vi "PLAN_CREATOR.vi"(8 "error In":errorcluster) -> (0 "error out":errorcluster)   [LabVIEW 2017]
uses:
  Controls/Ass. Loop Control.ctl
  <vilib>/Utility/error.llb/DialogType.ctl
panel:
  in  "PLAN NAME":string(combo)
  in  "CURRENT PLAN TABLE":string[][](table)
  in  "REMOVE PART":bool
  in  "ADD PART":bool
  in  "LIST OF PARTS":string(combo)
  in  "DOORS":string(combo)
  out "USER:-":string
  in  "Stop":bool
  out "DATE/TIME":string
  out "Screen Name":string
  # "Nm"
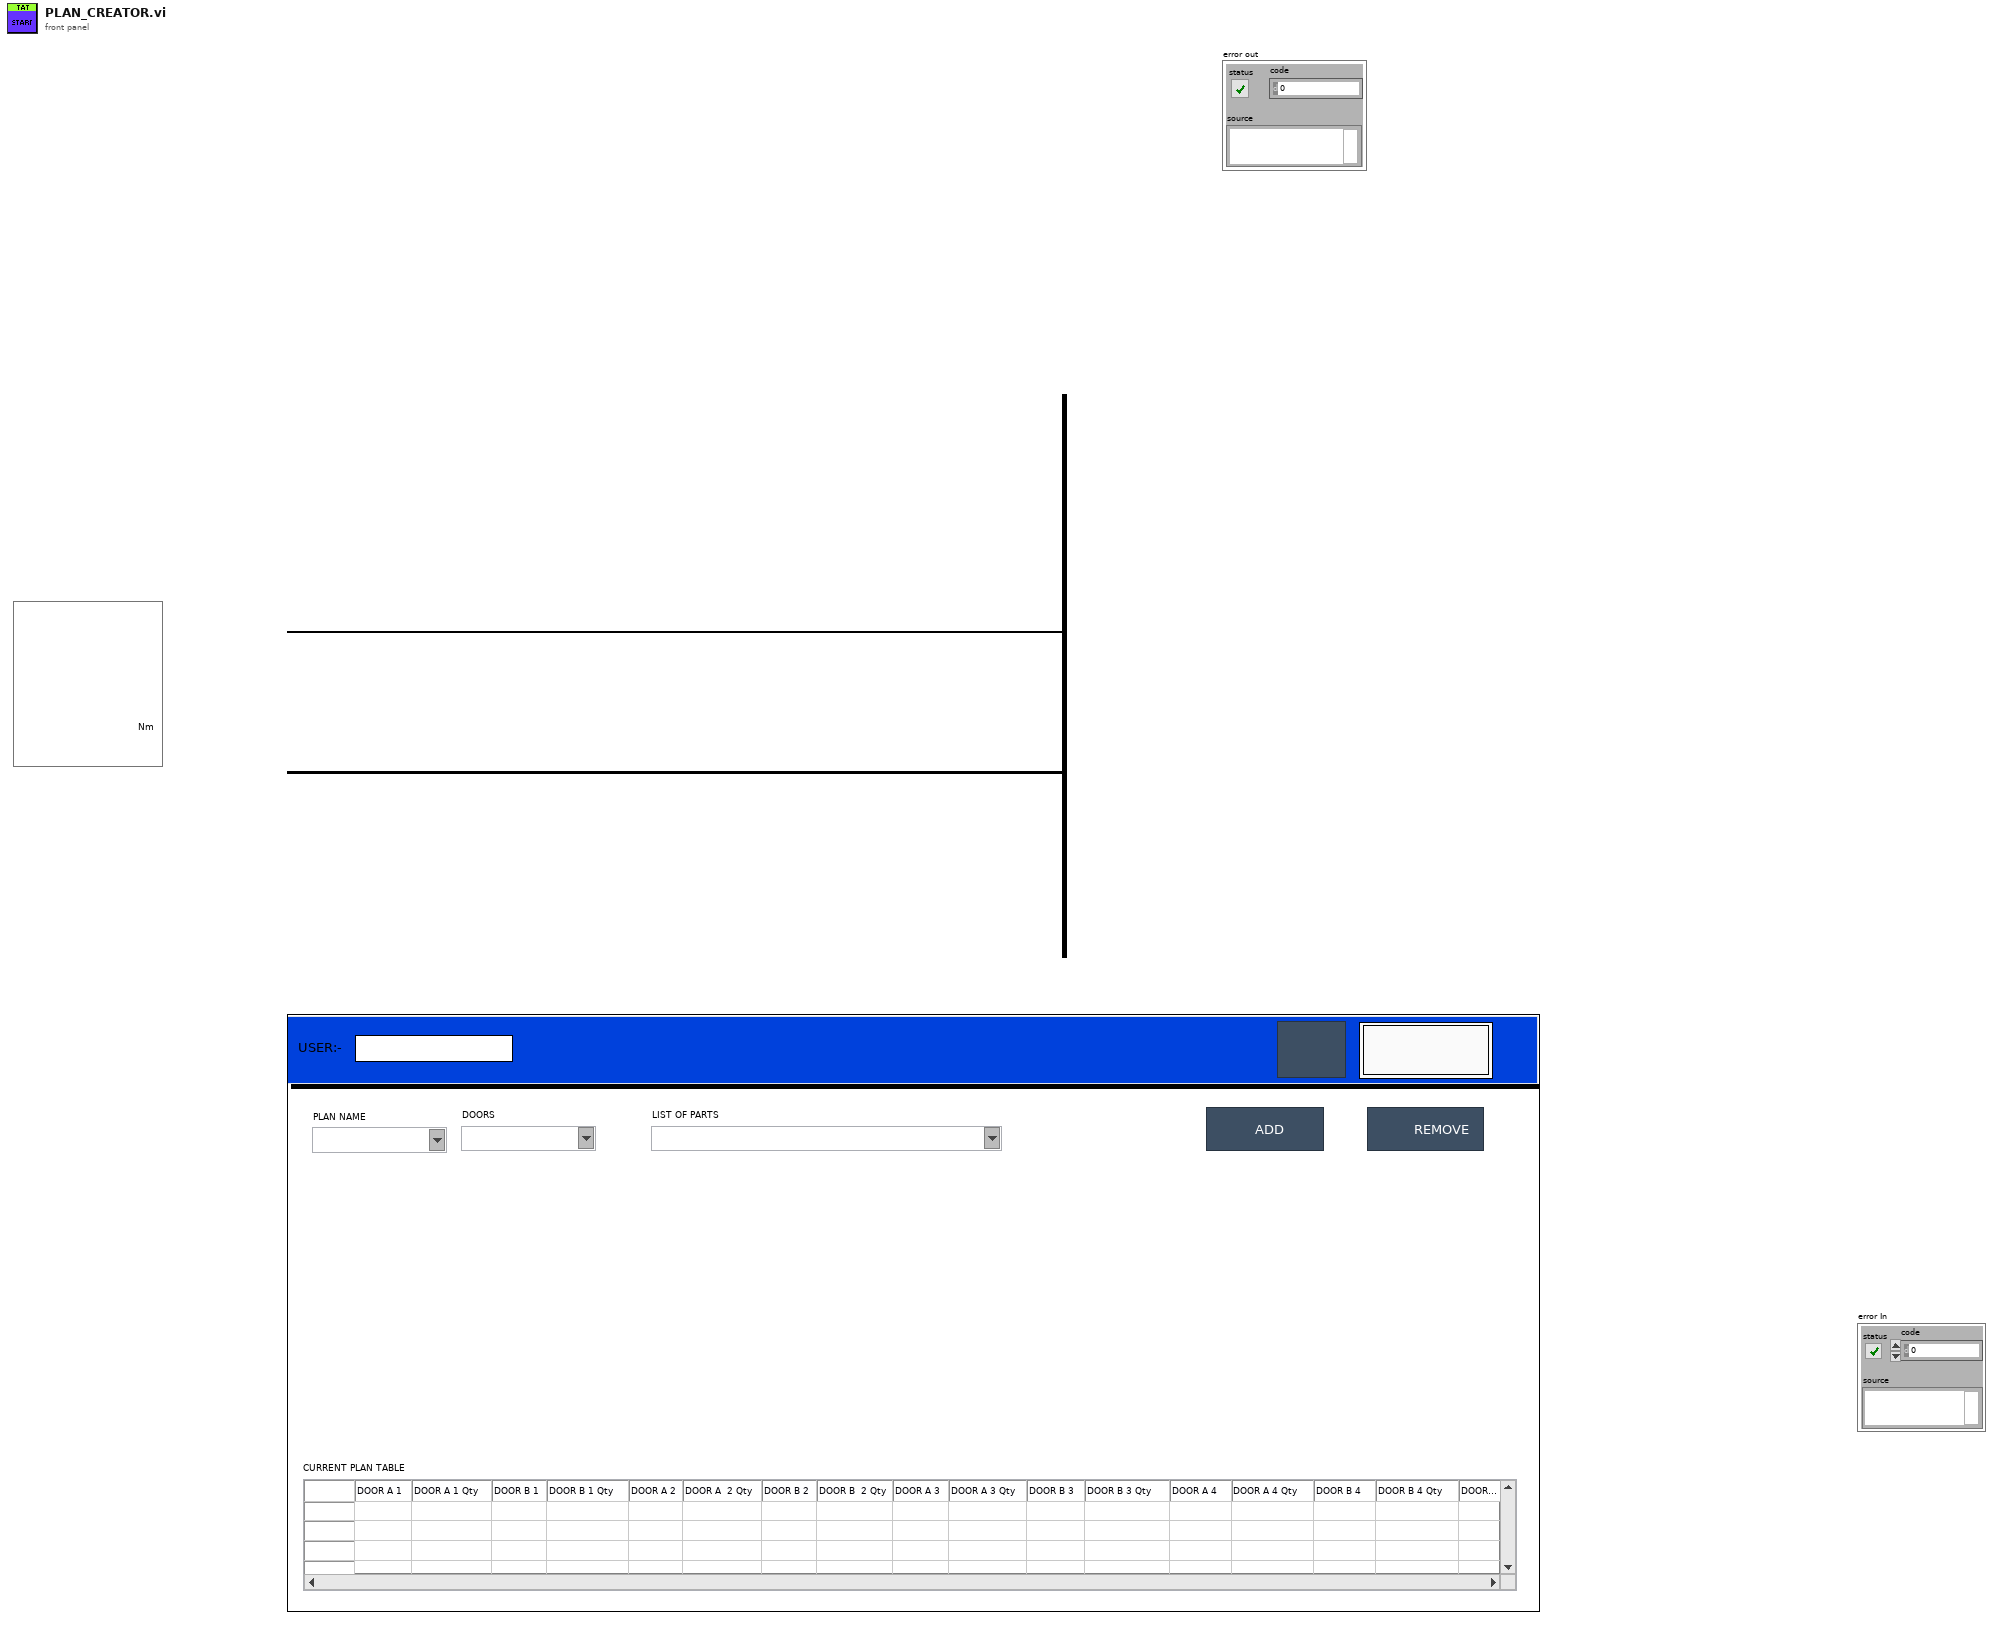
[diagram p1: front panel]
types:
  T1 = typedef "DialogType.ctl" = u16
  T2 = typedef "Ass. Loop Control.ctl" = enum16{"Package_Qty_Count", "GENERATE_QR_PRNT", "Cluster_update", "Waiting_for_scan", "barcode CHECK", "Int", "SaveReport ", "Barcode Print", "Start Cycle", "Wait", "Cycle End", "Stop"}
  T3 = enum32{"invalid app kind", "Development System", "Run Time System", "Student Edition", "Embedded LabVIEW", "Evaluation", "Custom"}
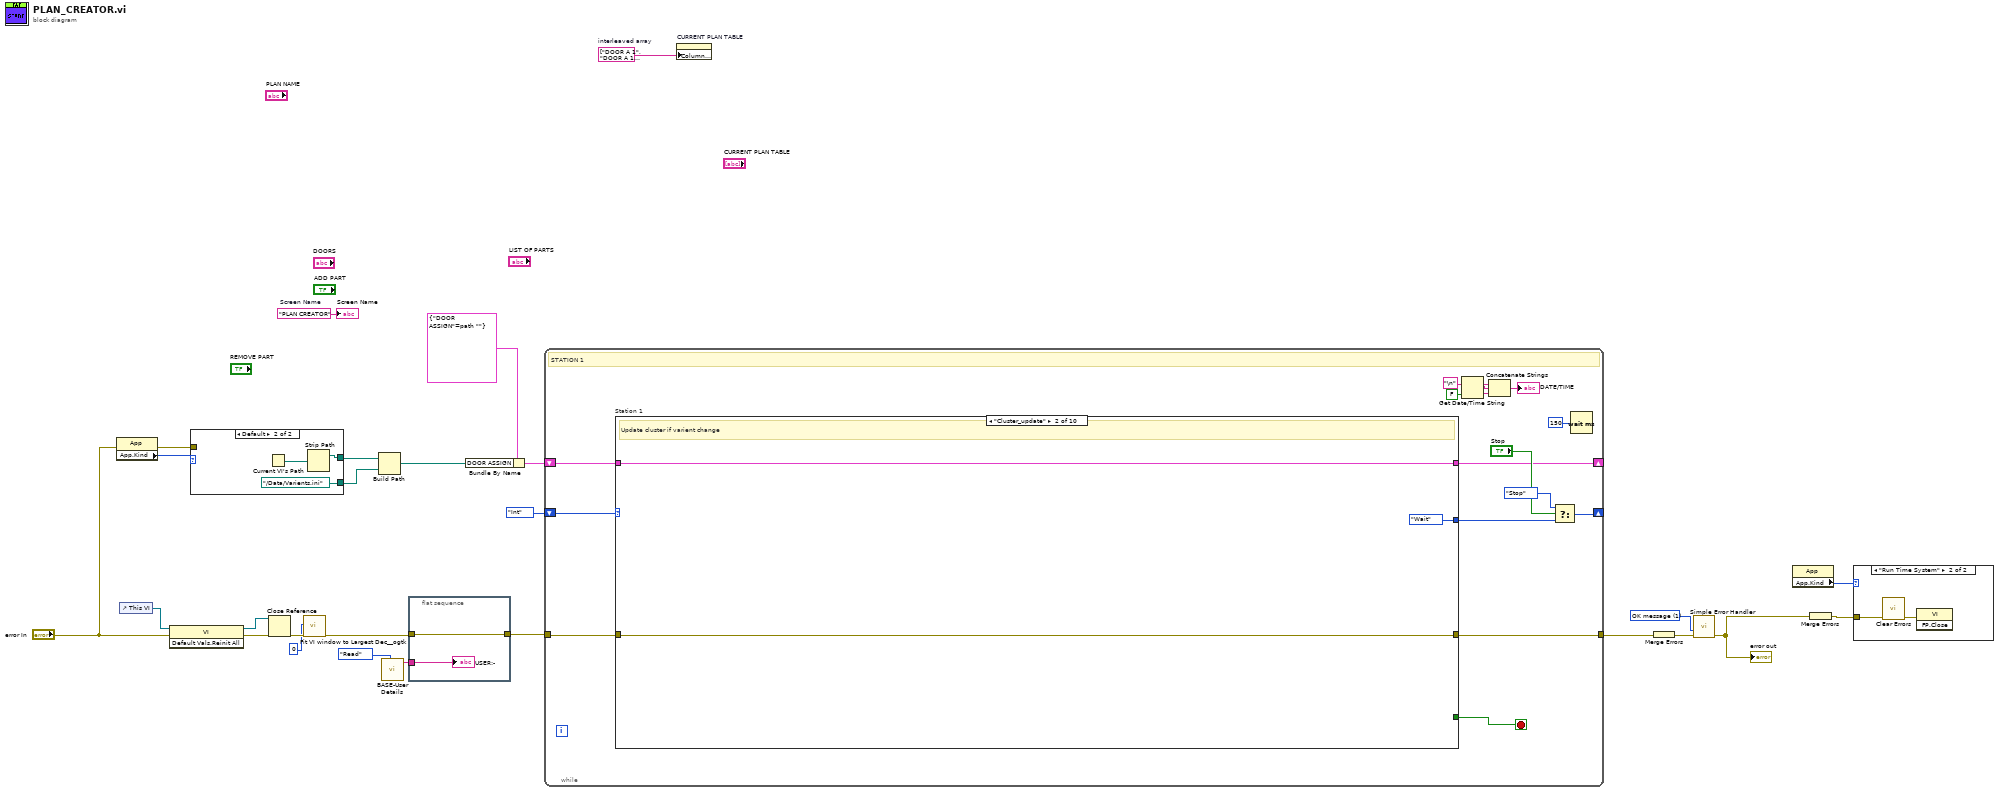
[diagram p0: block diagram]
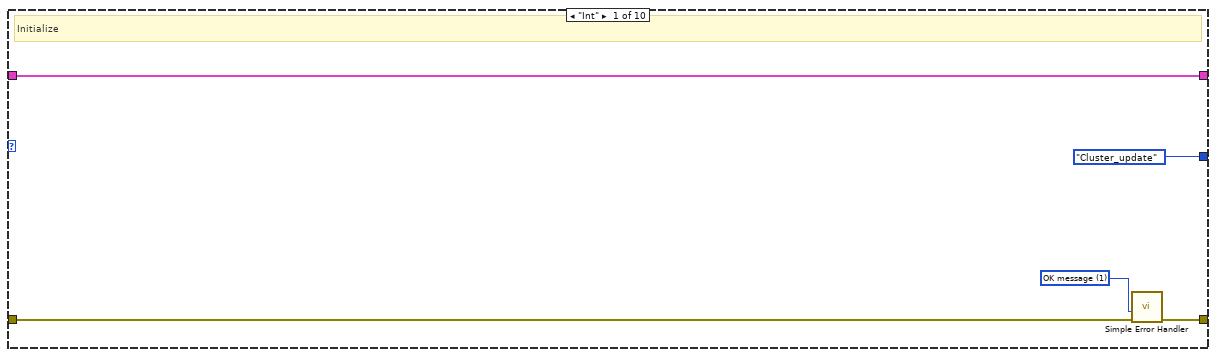
[diagram p3: hidden frame]
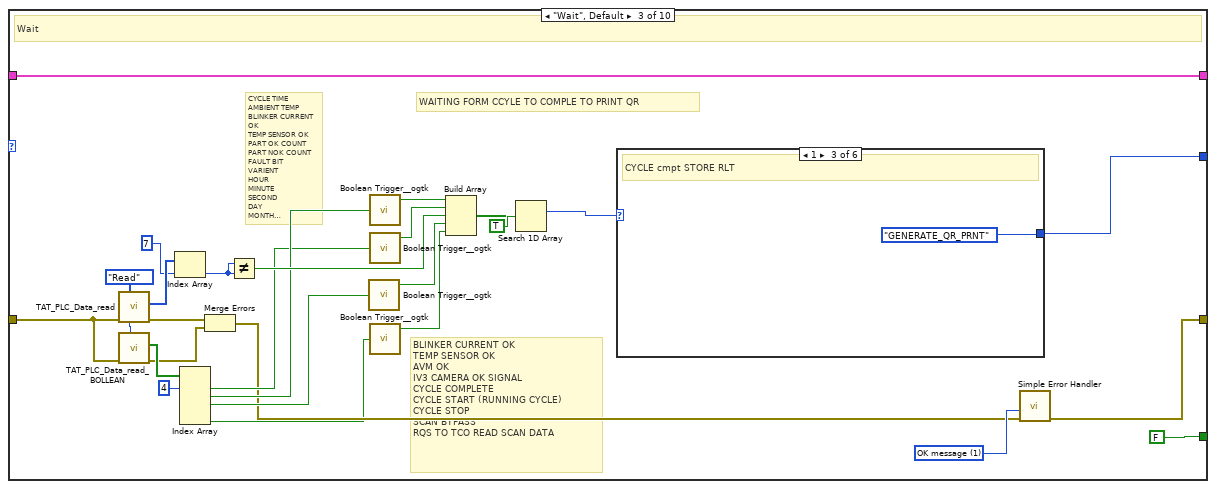
[diagram p4: hidden frame]
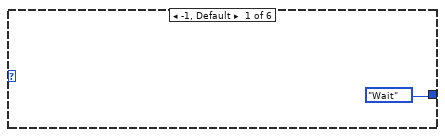
[diagram p5: hidden frame]
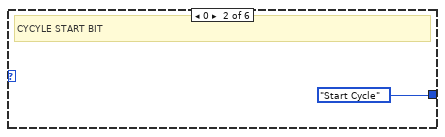
[diagram p6: hidden frame]
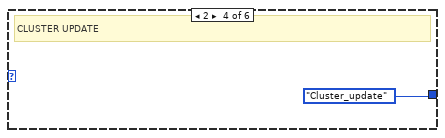
[diagram p7: hidden frame]
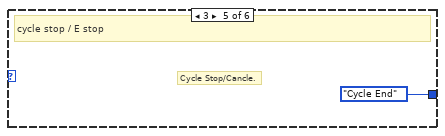
[diagram p8: hidden frame]
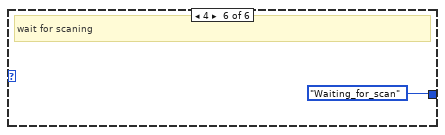
[diagram p9: hidden frame]
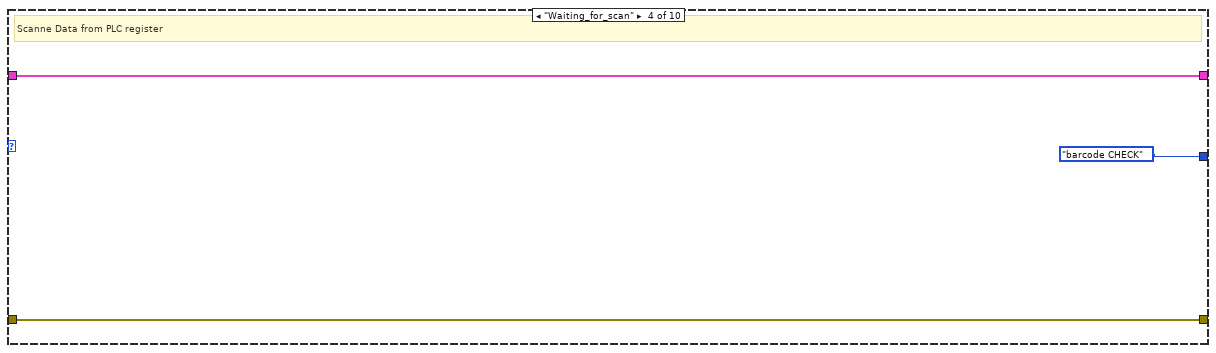
[diagram p10: hidden frame]
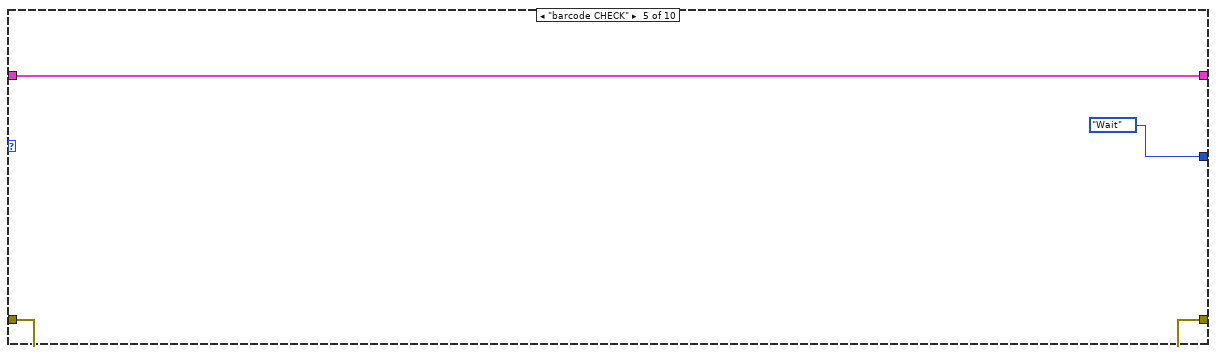
[diagram p11: hidden frame]
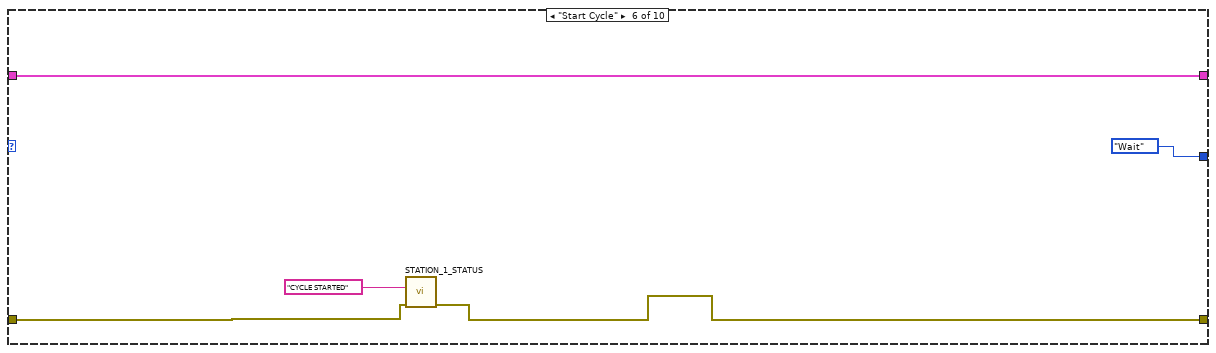
[diagram p12: hidden frame]
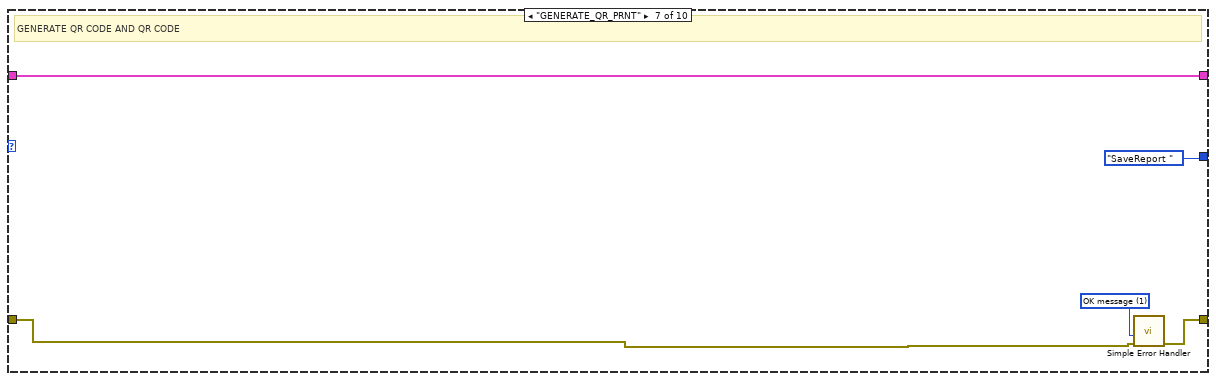
[diagram p13: hidden frame]
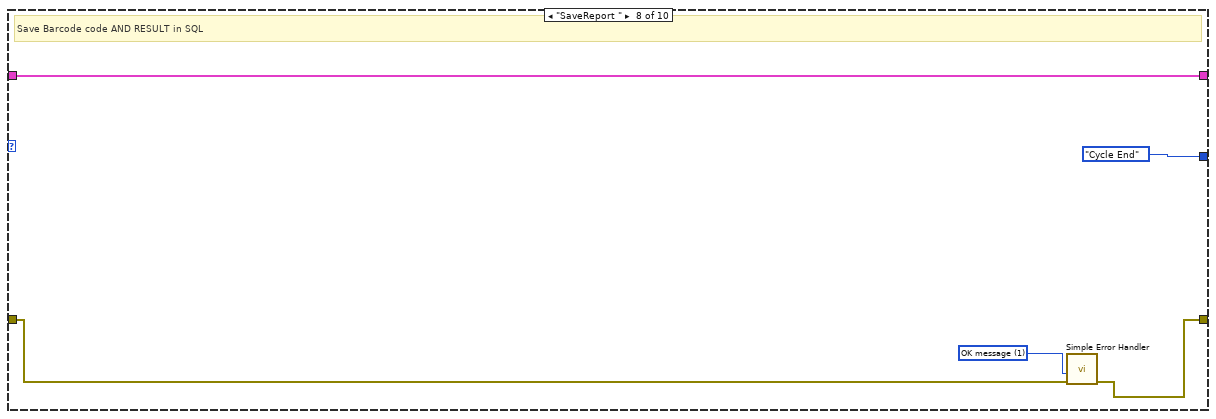
[diagram p14: hidden frame]
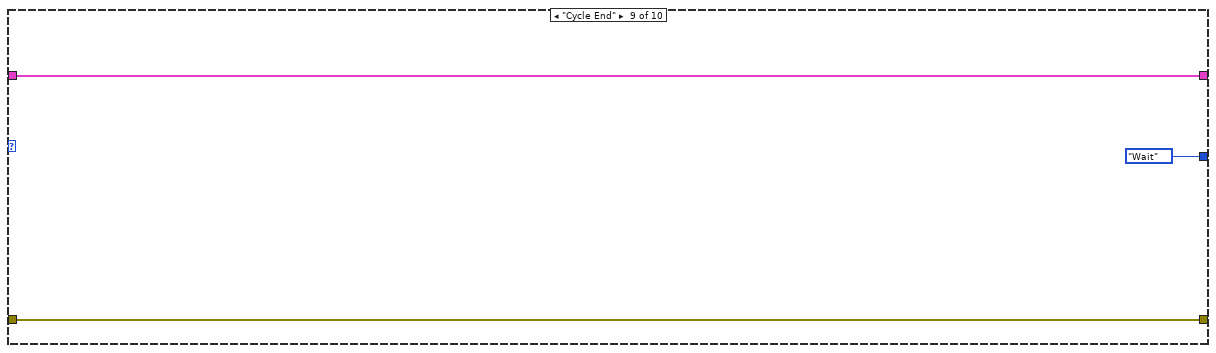
[diagram p15: hidden frame]
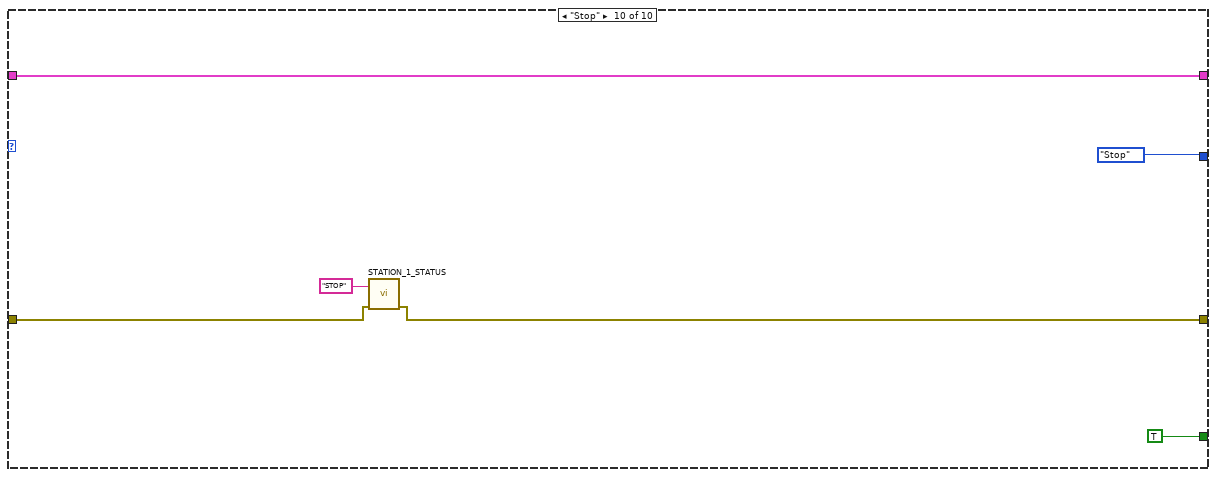
[diagram p16: hidden frame]
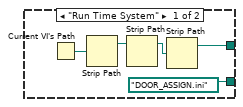
[diagram p17: hidden frame]
diagram:
  w1 = string[] ["DOOR A 1", "DOOR A 1 Qty", "DOOR B 1", "DOOR B 1 Qty", "DOOR A 2", "DOOR A  2 Qty", "DOOR B 2", "DOOR B  2 Qty", "DOOR A 3", "DOOR A 3 Qty", "DOOR B 3", "DOOR B 3 Qty", "DOOR A 4", "DOOR A 4 Qty", "DOOR B 4", "DOOR B 4 Qty", "DOOR A 5", "DOOR A 5 Qty", "DOOR B 5", "DOOR B 5 Qty", "DOOR A 11", "DOOR A 11 Qty", "DOOR B 11", "DOOR B 11 Qty", "DOOR A 12", "DOOR A 12 Qty", "DOOR B 12", "DOOR B 12 Qty", "DOOR A 13", "DOOR A 13 Qty", "DOOR B 13", "DOOR B 13 Qty", "DOOR A 14", "DOOR A 14 Qty", "DOOR B 14", "DOOR B 14 Qty", "DOOR A 15", "DOOR A 15 Qty", "DOOR B 15", "DOOR B 15 Qty", "DOOR A 16", "DOOR A 16 Qty", "DOOR B 16", "DOOR B 16 Qty"]  # interleaved array
  w5 = "PLAN CREATOR"  # Screen Name
  w17 = T1 1 items=["no dialog", "OK message", "continue or stop message", "OK message + warnings", "continue/stop + warnings"] ("type of dialog (OK msg:1)")
  n1 = property class="App"(error in="error In") -> (error out=w13:errorcluster, "App.Kind"=w15:T3)  [unwired: 1 in, 1 out]
  n2 = control-ref of="This VI"() -> (w26:refnum<vi>)
  n3 = invoke class="VI" method="Default Vals.Reinit All"(reference=w26, error in="error In") -> (reference out=w24:refnum<vi>, error out=w25:errorcluster)  [unwired: 1 in, 1 out]
  n4 = case shown="Default" w15 {
    tunnel: [path "DOOR_ASSIGN.ini" ("path") path "../Data/Varients.ini" ("path")] -> w14
    tunnel: [w27 w32] -> w7
    tunnel: w13 -> [_ _]
    frame "Run Time System" {
      n5 = Current VI's Path() -> (path=w30:path)
      n6 = Strip Path(path=w30) -> (stripped path=w29:path)  [unwired: 1 out]
      n7 = Strip Path(path=w29) -> (stripped path=w28:path)  [unwired: 1 out]
      n8 = Strip Path(path=w28) -> (stripped path=w27:path)  [unwired: 1 out]
    }
    frame Default {
      n9 = Current VI's Path() -> (path=w33:path)
      n10 = Strip Path(path=w33) -> (stripped path=w32:path)  [unwired: 1 out]
    }
  }
  n11 = Close Reference(reference=w24, error in (no error)=w25) -> (error out=w23:errorcluster)
  n12 = call <userlib>:"Fit VI window to Largest Dec__ogtk.vi"("error in (no error)"=w23, "border spacing (2 px)"=0) -> ("error out"=w11:errorcluster)  [unwired: 4 in, 1 out]
  n13 = Build Path(base path=w7, name or relative path=w14) -> (appended path=w3:path)
  n14 = call "BASE-User Details.vi"("Enum"=enum16{"Read", "Write"}."Read") -> ("User Name Out"=w18:string)  [unwired: 9 in, 1 out]
  n15 = flat-sequence {
    tunnel: [w36] -> w6
    tunnel: w11 -> [w36]
    tunnel: w18 -> [w35]
    frame #0 {
      "USER:-" <- w35
    }
  }
  n16 = Bundle By Name(cluster=cluster{"DOOR ASSIGN":path} {"DOOR ASSIGN"=path ""}, "DOOR ASSIGN"=w3) -> (w2:cluster{"DOOR ASSIGN":path})
  n17 = while {
    tunnel: w6 -> [w39]
    shift-right: [w49] -> _
    shift-left: Ass._Loop_Control."Int" ("Enum") -> [w52]
    tunnel: [w50] -> w21
    shift-right: [w37] -> _
    shift-left: w2 -> [w38]
    stop <- w42 stop-if-true
    # "STATION 1"
    n18 = case "Station 1" shown="\"Cluster_update\"" w52 {
      tunnel: [Ass._Loop_Control."Cluster_update" ("Enum") Ass._Loop_Control."Wait" ("Enum") w81 Ass._Loop_Control."barcode CHECK" ("Enum") Ass._Loop_Control."Wait" ("Enum") Ass._Loop_Control."Wait" ("Enum") Ass._Loop_Control."SaveReport " ("Enum") Ass._Loop_Control."Cycle End" ("Enum") Ass._Loop_Control."Wait" ("Enum") Ass._Loop_Control."Stop" ("Enum")] -> w41
      tunnel: [_ _ FALSE _ _ _ _ _ _ TRUE] -> w42
      tunnel: [w55 w59 w78 w95 w98 w101 w108 w112 w116 w119] -> w50
      tunnel: w39 -> [w54 w59 w75 w95 w98 w102 w106 w111 w116 w120]
      tunnel: w38 -> [w53 w58 w61 w94 w97 w100 w105 w110 w115 w118]
      tunnel: [w53 w58 w61 w94 w97 w100 w105 w110 w115 w118] -> w37
      frame "Int" {
        w56 = T1 1 items=["no dialog", "OK message", "continue or stop message", "OK message + warnings", "continue/stop + warnings"] ("type of dialog (OK msg:1)")
        # "Initialize"
        n19 = call <vilib>:"Simple Error Handler.vi"("type of dialog (OK msg:1)"=w56, "error in (no error)"=w54) -> ("error out"=w55:errorcluster)  [unwired: 3 in, 4 out]
      }
      frame "Cluster_update" {
        # "Update cluster if varient change"
      }
      frame "Wait", Default {
        w79 = T1 1 items=["no dialog", "OK message", "continue or stop message", "OK message + warnings", "continue/stop + warnings"] ("type of dialog (OK msg:1)")
        w76 = enum16{"Read", "Write"}."Read" ("Enum")
        # "CYCLE TIME\nAMBIENT TEMP\nBLINKER CURRENT OK\nTEMP SENSOR OK\nPART OK COUNT\nPART NOK COUNT\nFAULT BIT\nVARIENT\nHOUR\nMINUTE\nSECOND\nDAY\nMONTH\nYEAR\nSERIAL NUMBER"
        # "BLINKER CURRENT OK\nTEMP SENSOR OK\nAVM OK\nIV3 CAMERA OK SIGNAL\nCYCLE COMPLETE\nCYCLE START (RUNNING CYCLE)\nCYCLE STOP\nSCAN BYPASS\nRQS TO TCO READ SCAN DATA"
        # "WAITING FORM CCYLE TO COMPLE TO PRINT QR"
        # "Wait"
        n20 = call "TAT_PLC_Data_read.vi"("Enum"=w76, "error in (no error)"=w75) -> ("error out"=w66:errorcluster, "Array 2"=w82:u16[])  [unwired: 8 in]
        n21 = call "TAT_PLC_Data_read_BOLLEAN.vi"("Enum"=w76, "error in (no error)"=w75) -> ("error out"=w64:errorcluster, "Array 2"=w74:bool[])  [unwired: 8 in]
        n22 = Index Array(array=w82, index=7) -> (element=w62:u16)
        n23 = Index Array(array=w74, index #1=4 ("index")) -> (element #1=w71:bool, element #2=w72:bool, element #3=w70:bool, element #5=w63:bool)  [unwired: 4 in, 1 out]
        n24 = Merge Errors(w66, w64) -> (w65:errorcluster)
        n25 = Not Equal?(x=w62, y=w62) -> (x != y?=w80:bool)
        n26 = call <userlib>:"Boolean Trigger__ogtk.vi"("Boolean Input"=w70) -> ("Rising Edge"=w69:bool)  [unwired: 1 in, 1 out]
        n27 = call <userlib>:"Boolean Trigger__ogtk.vi"("Boolean Input"=w72) -> ("Rising Edge"=w86:bool)  [unwired: 1 in, 1 out]
        n28 = call <userlib>:"Boolean Trigger__ogtk.vi"("Boolean Input"=w71) -> ("Rising Edge"=w77:bool)  [unwired: 1 in, 1 out]
        n29 = call <userlib>:"Boolean Trigger__ogtk.vi"("Boolean Input"=w63) -> ("Rising Edge"=w68:bool)  [unwired: 1 in, 1 out]
        n30 = Build Array(w86, w77, w80, w69, w68) -> (w85:bool[])
        n31 = Search 1D Array(1D array=w85, element=TRUE ("Boolean Input")) -> (index of element=w84:i32)  [unwired: 1 in]
        n32 = case shown="1" w84 {
          tunnel: [Ass._Loop_Control."Wait" ("Enum") Ass._Loop_Control."Start Cycle" ("Enum") Ass._Loop_Control."GENERATE_QR_PRNT" ("Enum") Ass._Loop_Control."Cluster_update" ("Enum") Ass._Loop_Control."Cycle End" ("Enum") Ass._Loop_Control."Waiting_for_scan" ("Enum")] -> w81
          frame -1, Default {
          }
          frame 0 {
            # "CYCYLE START BIT"
          }
          frame 1 {
            # "CYCLE cmpt STORE RLT"
          }
          frame 2 {
            # "CLUSTER UPDATE"
          }
          frame 3 {
            # "Cycle Stop/Cancle."
            # "cycle stop / E stop"
          }
          frame 4 {
            # "wait for scaning"
          }
        }
        n33 = call <vilib>:"Simple Error Handler.vi"("type of dialog (OK msg:1)"=w79, "error in (no error)"=w65) -> ("error out"=w78:errorcluster)  [unwired: 3 in, 4 out]
      }
      frame "Waiting_for_scan" {
        # "Scanne Data from PLC register"
      }
      frame "barcode CHECK" {
      }
      frame "Start Cycle" {
        n34 = call "STATION_1_STATUS.vi"("error in (no error)"=w102, "STATUS"="CYCLE STARTED" ("Cycle Status")) -> ("error out"=w101:errorcluster)  [unwired: 9 in]
      }
      frame "GENERATE_QR_PRNT" {
        w109 = T1 1 items=["no dialog", "OK message", "continue or stop message", "OK message + warnings", "continue/stop + warnings"] ("type of dialog (OK msg:1)")
        # "GENERATE QR CODE AND QR CODE"
        n35 = call <vilib>:"Simple Error Handler.vi"("type of dialog (OK msg:1)"=w109, "error in (no error)"=w106) -> ("error out"=w108:errorcluster)  [unwired: 3 in, 4 out]
      }
      frame "SaveReport " {
        w113 = T1 1 items=["no dialog", "OK message", "continue or stop message", "OK message + warnings", "continue/stop + warnings"] ("type of dialog (OK msg:1)")
        # "Save Barcode code AND RESULT in SQL"
        n36 = call <vilib>:"Simple Error Handler.vi"("type of dialog (OK msg:1)"=w113, "error in (no error)"=w111) -> ("error out"=w112:errorcluster)  [unwired: 3 in, 4 out]
      }
      frame "Cycle End" {
      }
      frame "Stop" {
        n37 = call "STATION_1_STATUS.vi"("error in (no error)"=w120, "STATUS"="STOP" ("Cycle Status")) -> ("error out"=w119:errorcluster)  [unwired: 9 in]
      }
    }
    n38 = Get Date/Time String(want seconds? (F)=FALSE) -> (date string=w46:string, time string=w45:string)  [unwired: 2 in]
    n39 = Concatenate Strings(w46, "\n", w45) -> (→"DATE/TIME":string)
    n40 = Select(t=Ass._Loop_Control."Stop" ("Enum"), s="Stop", f=w41) -> (s? t:f=w49:T2)
    n41 = Wait (ms)(milliseconds to wait=u32 150) -> ()  [unwired: 1 out]
  }
  n42 = property on="CURRENT PLAN TABLE" class="Tbl (strict)"("Column Headers[]"=w1) -> ()  [unwired: 2 in, 2 out]
  n43 = Merge Errors(w21) -> (w20:errorcluster)
  n44 = call <vilib>:"Simple Error Handler.vi"("type of dialog (OK msg:1)"=w17, "error in (no error)"=w20) -> ("error out"=w8:errorcluster)  [unwired: 3 in, 4 out]
  "error out" <- w8
  n45 = property class="App"() -> ("App.Kind"=w16:T3)  [unwired: 2 in, 2 out]
  n46 = Merge Errors(w8) -> (w9:errorcluster)
  n47 = case shown="\"Run Time System\"" w16 {
    tunnel: w9 -> [_ w125]
    frame "invalid app kind", Default {
    }
    frame "Run Time System" {
      n48 = call <vilib>:"Clear Errors.vi"("error in (no error)"=w125) -> ("error out"=w124:errorcluster)  [unwired: 5 in, 1 out]
      n49 = invoke class="VI" method="FP.Close"(error in=w124) -> ()  [unwired: 2 in, 3 out]
    }
  }
  "Screen Name" <- w5
